vi "Exposure Time.vi"(11 "Test Case In":refnum<class "Test.Camera.lvclass">) -> (0 "error out":errorcluster, 3 "Test Case Out":refnum<class "Test.Camera.lvclass">)   [LabVIEW 2020, in "Test.Camera.lvclass"]
uses:
  Test.Camera.lvclass
  C:/Program Files (x86)/National Instruments/LabVIEW 2020/vi.lib/Astemes/LUnit/Test Case.lvclass
  g_industrial_cam/Camera/Camera.lvclass/Camera.ctl
  <vilib>/Astemes/LUnit/Test Case.lvclass/Test Case.ctl
  g_industrial_cam/Camera/Auto Mode.ctl
  c3e2611f-c54f-4219-a549-b8da21c7f085.vi
  0aa1576c-e916-4ad0-9a97-64bd3e4eb69b.vi
  1bd7569c-e4e0-4b2a-9900-dc183130fa42.vi
  35212a07-d7d8-4da5-a00d-57064e45d28a.vi
  g_industrial_cam/Camera/GetSetExposureTime.vi
  g_industrial_cam/Camera/GetSetExposureTimeAuto.vi
  <vilib>/Astemes/LUnit/Append Pass Result.vi
  <vilib>/Astemes/LUnit/Append Fail Result.vi
  <vilib>/Astemes/LUnit/Describe Comparison.vi
  0aa1576c-e916-4ad0-9a97-64bd3e4eb69b.vi/9c5d11cd-9439-4240-a1ee-d9baace9c924.vi
  45f0f70e-dc75-4703-ae84-689abf371a5e.vi/23ce184e-9622-4817-bac2-1c972340de52.vi
  45f0f70e-dc75-4703-ae84-689abf371a5e.vi/3848369b-d3fa-48af-9fdc-8c3f580b91af.vi
  1bd7569c-e4e0-4b2a-9900-dc183130fa42.vi/9c5d11cd-9439-4240-a1ee-d9baace9c924.vi
  g_industrial_cam/Camera/Get Value (String).vi
  g_industrial_cam/Camera/Get Exposure Mode.vi/1d0181f0-64a9-471c-9d08-be33338c9a07.vi
  g_industrial_cam/Camera/Get Exposure Mode.vi/84d87f68-00df-4f07-8889-951d30b90fde.vi
  fc55cd85-1f0e-4836-bb3d-02d21993f554.vi/23ce184e-9622-4817-bac2-1c972340de52.vi
  fc55cd85-1f0e-4836-bb3d-02d21993f554.vi/3848369b-d3fa-48af-9fdc-8c3f580b91af.vi
  35212a07-d7d8-4da5-a00d-57064e45d28a.vi/9c5d11cd-9439-4240-a1ee-d9baace9c924.vi
  <vilib>/Astemes/LUnit/Run In UI.vi
  g_industrial_cam/Camera/GetSetStringValue.vi
  <vilib>/Utility/error.llb/Clear Errors.vi
  g_industrial_cam/Camera/Check Not Disconnected.vi
  <vilib>/Utility/error.llb/Error Cluster From Error Code.vi
  <vilib>/Astemes/LUnit/Describe Variant.vi
  <vilib>/Comparison/Equal/Equal Functor/Equal Functor.lvclass
  Test.Camera.lvclass/Test.Camera.ctl
  <vilib>/Astemes/LUnit/Test Case.lvclass
  g_industrial_cam/Camera/Camera.lvclass
  c945e279-9ae8-4d86-b97f-5f20c85afebd.vi
  4ff0574b-22d9-4cf5-8c1e-dfd5ab83d1de.vi
  C:/Program Files (x86)/National Instruments/LabVIEW 2020/vi.lib/Astemes/LUnit/LUnit Runnable.lvclass
  C:/serenial/lib/g-industrial-camera/LabVIEW/tests/Test.Camera/Test.Camera.lvclass
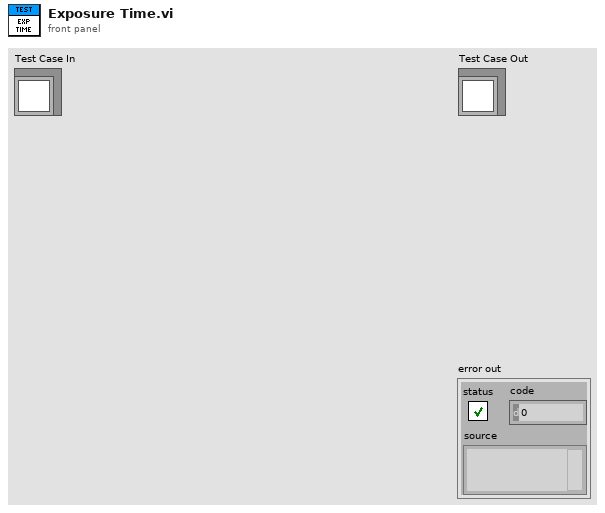
[diagram p1: front panel]
types:
  T1 = enum16{"Get Values", "Set Exposure", "Set Auto Exposure", "Set Exposure Mode"}
  T2 = typedef "Camera.lvclass/Auto Mode.ctl" = enum8{"Off", "Once", "Continuous"}
  T3 = enum16{"Get Values", "Set Exposure", "Set Auto Exposure", "Set Exposure Mode"}[]
  T4 = typedef "Camera.lvclass/Exposure Mode.ctl" = enum8{"Off", "Timed", "Trigger Width", "Trigger Controller"}
  T5 = typedef "Camera.lvclass/Representation.ctl" = enum8{"Undefined", "Linear", "Logarithmic", "Boolean", "Pure Number", "Hex Number", "IP Address", "MAC Address"}
  T6 = cluster{"Auto Mode":T2, "Auto Avaliable":bool, "Representation":T5, "Min (us)":dbl, "Max (us)":dbl, "Time (us)":dbl, "Exposure Time Available":bool, "Exposure Modes":T4[], "Exposure Mode":T4}
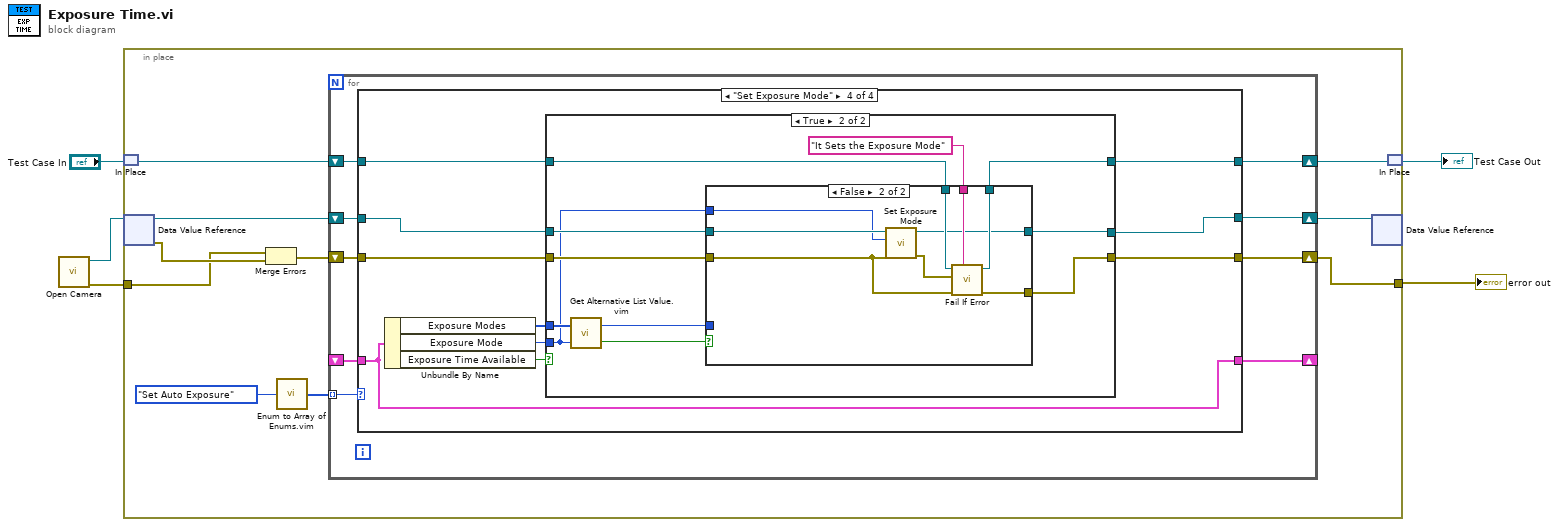
[diagram p0: block diagram]
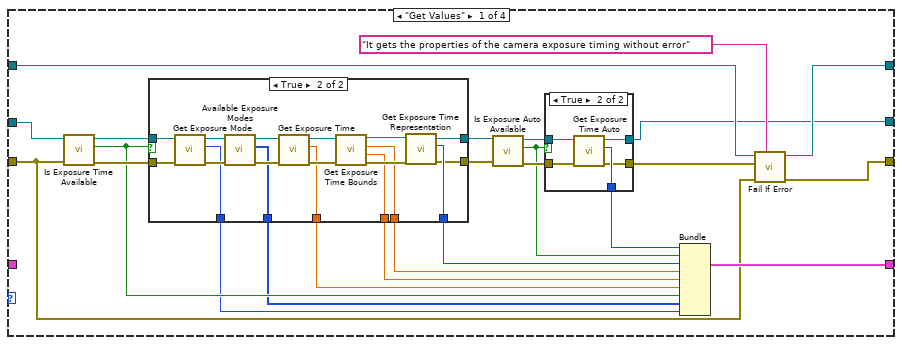
[diagram p2: hidden frame]
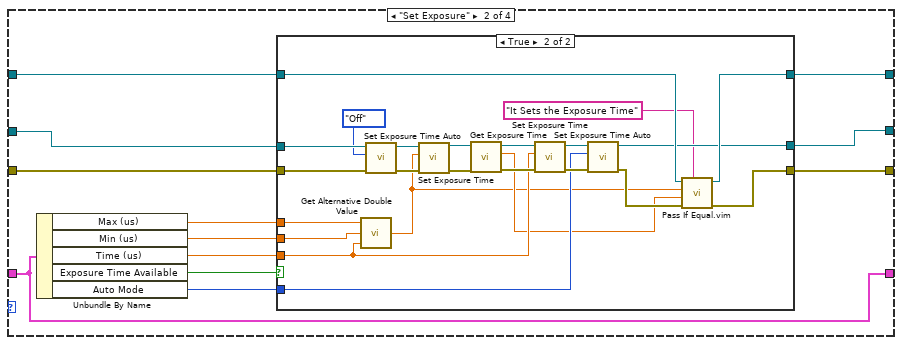
[diagram p5: hidden frame]
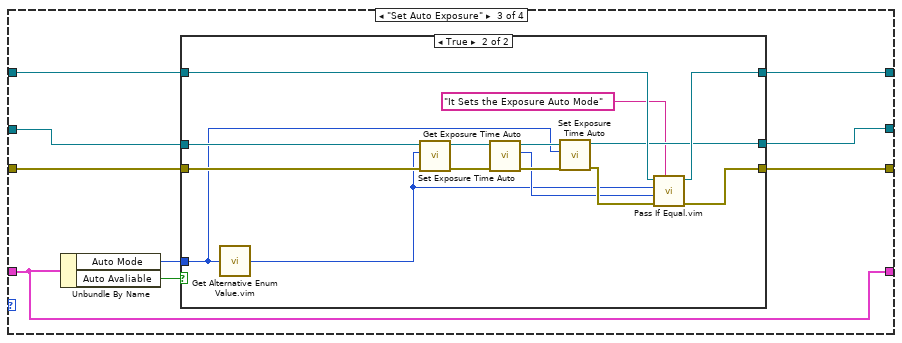
[diagram p7: hidden frame]
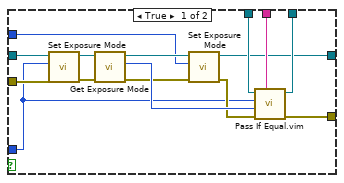
[diagram p10: hidden frame]
diagram:
  n1 = call "Open Camera.vi"() -> ("error out"=w5:errorcluster, "Camera"=w4:refnum<data-value>)  [unwired: 10 in]
  n2 = in-place {
    in-place-border: w5 -> [w8]
    in-place-border: [w7] -> w2
    n3 = in-place-match #1("Test Case In") -> (w10:refnum<class "Test.Camera.lvclass">)
    n4 = in-place-dvr #2(w4) -> (w14:refnum<class "Camera.lvclass">, w15:errorcluster)
    n5 = Merge Errors(w8, w15) -> (w13:errorcluster)
    n6 = call "Enum to Array of Enums.vim"("enum"=T1."Set Auto Exposure") -> ("array of enums"=w11:T3)
    n7 = for {
      tunnel: w11 -> [w22] mode=indexing
      shift-right: [w21] -> w9
      shift-left: w14 -> [w24]
      shift-right: [w20] -> _
      shift-left: _ -> [w19]
      shift-right: [w17] -> w6
      shift-left: w10 -> [w18]
      shift-right: [w16] -> w7
      shift-left: w13 -> [w23]
      n8 = case shown="\"Set Exposure Mode\"" w22 {
        tunnel: w24 -> [w43 w86 w121 w149]
        tunnel: w23 -> [w42 w87 w122 w150]
        tunnel: [w28 w78 w117 w145] -> w21
        tunnel: [w44 w76 w115 w143] -> w20
        tunnel: w19 -> [_ w76 w115 w143]
        tunnel: w18 -> [w48 w80 w119 w147]
        tunnel: [w47 w79 w118 w146] -> w17
        tunnel: [w45 w77 w116 w144] -> w16
        frame "Get Values" {
          n9 = call "Is Exposure Time Available.vi"("error in (no error)"=w42, "Camera in"=w43) -> ("error out"=w41:errorcluster, "Exposure Time Available"=w40:bool, "Camera"=w39:refnum<class "Camera.lvclass">)  [unwired: 7 in]
          n10 = case shown="True" w40 {
            tunnel: w41 -> [w56 w75]
            tunnel: w39 -> [w57 w60]
            tunnel: [_ w70] -> w38
            tunnel: [_ w69] -> w37
            tunnel: [_ w68] -> w36
            tunnel: [_ w67] -> w35
            tunnel: [w56 w66] -> w34
            tunnel: [w57 w65] -> w33
            tunnel: [_ w62] -> w26
            tunnel: [_ w58] -> w25
            frame False {
            }
            frame True {
              n11 = call "Get Exposure Mode.vi"("error in (no error)"=w75, "Camera in"=w60) -> ("error out"=w61:errorcluster, "Exposure Mode"=w58:T4, "Camera"=w59:refnum<class "Camera.lvclass">)  [unwired: 7 in]
              n12 = call "Available Exposure Modes.vi"("error in (no error)"=w61, "Camera in"=w59) -> ("error out"=w64:errorcluster, "Exposure Modes"=w62:T4[], "Camera"=w63:refnum<class "Camera.lvclass">)  [unwired: 7 in]
              n13 = call "Get Exposure Time.vi"("error in (no error)"=w64, "Camera in"=w63) -> ("error out"=w74:errorcluster, "Time (us)"=w70:dbl, "Camera"=w73:refnum<class "Camera.lvclass">)  [unwired: 7 in]
              n14 = call "Get Exposure Time Bounds.vi"("error in (no error)"=w74, "Camera in"=w73) -> ("error out"=w72:errorcluster, "Max (us)"=w69:dbl, "Min (us)"=w68:dbl, "Camera"=w71:refnum<class "Camera.lvclass">)  [unwired: 6 in]
              n15 = call "Get Exposure Time Representation.vi"("error in (no error)"=w72, "Camera in"=w71) -> ("error out"=w66:errorcluster, "Representation"=w67:T5, "Camera"=w65:refnum<class "Camera.lvclass">)  [unwired: 7 in]
            }
          }
          n16 = call "Is Exposure Auto Available.vi"("error in (no error)"=w34, "Camera in"=w33) -> ("error out"=w32:errorcluster, "Auto Avaliable"=w30:bool, "Camera"=w31:refnum<class "Camera.lvclass">)  [unwired: 7 in]
          n17 = case shown="True" w30 {
            tunnel: w32 -> [w50 w55]
            tunnel: w31 -> [w49 w54]
            tunnel: [_ w53] -> w29
            tunnel: [w49 w52] -> w28
            tunnel: [w50 w51] -> w27
            frame False {
            }
            frame True {
              n18 = call "Get Exposure Time Auto.vi"("error in (no error)"=w55, "Camera in"=w54) -> ("error out"=w51:errorcluster, "Auto Mode"=w53:T2, "Camera"=w52:refnum<class "Camera.lvclass">)  [unwired: 7 in]
            }
          }
          n19 = Bundle("Auto Mode"=w29, "Auto Avaliable"=w30, "Representation"=w35, "Min (us)"=w36, "Max (us)"=w37, "Time (us)"=w38, "Exposure Time Available"=w40, "Exposure Modes"=w26, "Exposure Mode"=w25) -> (w44:T6)  [unwired: 1 in]
          n20 = call <vilib>:"Fail If Error.vi"("Description"="It gets the properties of the camera exposure timing without error", "error in (no error)"=w42, "Assert error"=w27, "LUnit Test Case In"=w48) -> ("error out"=w45:errorcluster, "LUnit Test Case Out"=w47:refnum<class "Test.Camera.lvclass">)  [unwired: 6 in]
        }
        frame "Set Exposure" {
          n21 = Unbundle By Name(w76) -> ("Max (us)"=w84:dbl, "Min (us)"=w83:dbl, "Time (us)"=w82:dbl, "Exposure Time Available"=w85:bool, "Auto Mode"=w81:T2)
          n22 = case shown="True" w85 {
            tunnel: w87 -> [w90 w113]
            tunnel: w86 -> [w89 w111]
            tunnel: w84 -> [_ w108]
            tunnel: w83 -> [_ w107]
            tunnel: w82 -> [_ w102]
            tunnel: w81 -> [_ w100]
            tunnel: w80 -> [w88 w98]
            tunnel: [w88 w97] -> w79
            tunnel: [w89 w95] -> w78
            tunnel: [w90 w94] -> w77
            frame False {
            }
            frame True {
              n23 = call "Get Alternative Double Value.vi"("Value"=w102, "Min"=w107, "Max"=w108) -> ("Alternative Value"=w91:dbl)  [unwired: 1 in]
              n24 = call "Set Exposure Time Auto.vi"("error in (no error)"=w113, "Mode"=Auto_Mode."Off", "Camera in"=w111) -> ("error out"=w112:errorcluster, "Camera"=w109:refnum<class "Camera.lvclass">)  [unwired: 7 in]
              n25 = call "Set Exposure Time.vi"("error in (no error)"=w112, "Time (us)"=w91, "Camera in"=w109) -> ("error out"=w106:errorcluster, "Camera"=w105:refnum<class "Camera.lvclass">)  [unwired: 7 in]
              n26 = call "Get Exposure Time.vi"("error in (no error)"=w106, "Camera in"=w105) -> ("error out"=w104:errorcluster, "Time (us)"=w92:dbl, "Camera"=w103:refnum<class "Camera.lvclass">)  [unwired: 7 in]
              n27 = call "Set Exposure Time.vi"("error in (no error)"=w104, "Time (us)"=w102, "Camera in"=w103) -> ("error out"=w101:errorcluster, "Camera"=w99:refnum<class "Camera.lvclass">)  [unwired: 7 in]
              n28 = call "Set Exposure Time Auto.vi"("error in (no error)"=w101, "Mode"=w100, "Camera in"=w99) -> ("error out"=w96:errorcluster, "Camera"=w95:refnum<class "Camera.lvclass">)  [unwired: 7 in]
              n29 = call "Pass If Equal.vim"("Description"="It Sets the Exposure Time", "error in (no error)"=w96, "Actual"=w92, "Expected"=w91, "LUnit Test Case In"=w98) -> ("error out"=w94:errorcluster, "LUnit Test Case Out"=w97:refnum<class "Test.Camera.lvclass">)  [unwired: 5 in]
            }
          }
        }
        frame "Set Auto Exposure" {
          n30 = Unbundle By Name(w115) -> ("Auto Mode"=w114:T2, "Auto Avaliable"=w120:bool)
          n31 = case shown="True" w120 {
            tunnel: w122 -> [w125 w140]
            tunnel: w121 -> [w124 w139]
            tunnel: w119 -> [w123 w137]
            tunnel: [w123 w136] -> w118
            tunnel: [w124 w134] -> w117
            tunnel: [w125 w133] -> w116
            tunnel: w114 -> [_ w126]
            frame False {
            }
            frame True {
              n32 = call "Get Alternative Enum Value.vim"("Enum In"=w126) -> ("Alternative Value"=w127:T2)
              n33 = call "Set Exposure Time Auto.vi"("error in (no error)"=w140, "Mode"=w127, "Camera in"=w139) -> ("error out"=w138:errorcluster, "Camera"=w130:refnum<class "Camera.lvclass">)  [unwired: 7 in]
              n34 = call "Get Exposure Time Auto.vi"("error in (no error)"=w138, "Camera in"=w130) -> ("error out"=w131:errorcluster, "Auto Mode"=w128:T2, "Camera"=w129:refnum<class "Camera.lvclass">)  [unwired: 7 in]
              n35 = call "Set Exposure Time Auto.vi"("error in (no error)"=w131, "Mode"=w126, "Camera in"=w129) -> ("error out"=w135:errorcluster, "Camera"=w134:refnum<class "Camera.lvclass">)  [unwired: 7 in]
              n36 = call "Pass If Equal.vim"("Description"="It Sets the Exposure Auto Mode", "error in (no error)"=w135, "Actual"=w128, "Expected"=w127, "LUnit Test Case In"=w137) -> ("error out"=w133:errorcluster, "LUnit Test Case Out"=w136:refnum<class "Test.Camera.lvclass">)  [unwired: 5 in]
            }
          }
        }
        frame "Set Exposure Mode" {
          n37 = Unbundle By Name(w143) -> ("Exposure Modes"=w142:T4[], "Exposure Mode"=w141:T4, "Exposure Time Available"=w148:bool)
          n38 = case shown="True" w148 {
            tunnel: w150 -> [w153 w158]
            tunnel: w149 -> [w152 w159]
            tunnel: w147 -> [w151 w164]
            tunnel: [w151 w163] -> w146
            tunnel: [w152 w160] -> w145
            tunnel: [w153 w162] -> w144
            tunnel: w142 -> [_ w157]
            tunnel: w141 -> [_ w155]
            frame False {
            }
            frame True {
              n39 = call "Get Alternative List Value.vim"("Current Value"=w155, "List in"=w157) -> ("Other Value Available"=w154:bool, "Other Value"=w156:T4)
              n40 = case shown="False" w154 {
                tunnel: w164 -> [w179 w188]
                tunnel: [w178 w187] -> w163
                tunnel: [w177 w186] -> w162
                tunnel: "It Sets the Exposure Mode" ("Description") -> [w176 w185]
                tunnel: [w169 w184] -> w160
                tunnel: w159 -> [w168 w183]
                tunnel: w158 -> [w167 w180]
                tunnel: w156 -> [w166 _]
                tunnel: w155 -> [w165 w182]
                frame True {
                  n41 = call "Set Exposure Mode.vi"("error in (no error)"=w167, "Exposure Mode"=w166, "Camera in"=w168) -> ("error out"=w175:errorcluster, "Camera"=w174:refnum<class "Camera.lvclass">)  [unwired: 7 in]
                  n42 = call "Get Exposure Mode.vi"("error in (no error)"=w175, "Camera in"=w174) -> ("error out"=w172:errorcluster, "Exposure Mode"=w173:T4, "Camera"=w171:refnum<class "Camera.lvclass">)  [unwired: 7 in]
                  n43 = call "Set Exposure Mode.vi"("error in (no error)"=w172, "Exposure Mode"=w165, "Camera in"=w171) -> ("error out"=w170:errorcluster, "Camera"=w169:refnum<class "Camera.lvclass">)  [unwired: 7 in]
                  n44 = call "Pass If Equal.vim"("Description"=w176, "error in (no error)"=w170, "Actual"=w173, "Expected"=w166, "LUnit Test Case In"=w179) -> ("error out"=w177:errorcluster, "LUnit Test Case Out"=w178:refnum<class "Test.Camera.lvclass">)  [unwired: 5 in]
                }
                frame False {
                  n45 = call "Set Exposure Mode.vi"("error in (no error)"=w180, "Exposure Mode"=w182, "Camera in"=w183) -> ("error out"=w181:errorcluster, "Camera"=w184:refnum<class "Camera.lvclass">)  [unwired: 7 in]
                  n46 = call <vilib>:"Fail If Error.vi"("Description"=w185, "error in (no error)"=w180, "Assert error"=w181, "LUnit Test Case In"=w188) -> ("error out"=w186:errorcluster, "LUnit Test Case Out"=w187:refnum<class "Test.Camera.lvclass">)  [unwired: 6 in]
                }
              }
            }
          }
        }
      }
    }
    n47 = in-place-dvr #2(w9) -> ()  [unwired: 2 out]
    n48 = in-place-match #1(w6) -> (→"Test Case Out":refnum<class "Test.Camera.lvclass">)
  }
  "error out" <- w2
